vi "Tell.vi"(4 "Priority":bool, 6 "Self Attributes":refnum<class "Attributes.lvclass">, 8 "Relation":T1, 9 "Msg":refnum<class "Msg.lvclass">, 10 "Address":refnum<user-event>) -> (0 "Error out":errorcluster)   [LabVIEW 2025, in "jettl.lvlib" / "Actor.lvlib"]
uses:
  Actor.lvlib
  Msg/Msg.lvclass
  Attributes/Attributes/Attributes.lvclass
  Relation.ctl
  <vilib>/event_ctls.llb/usereventprio.ctl
  Teller/Teller.lvlib
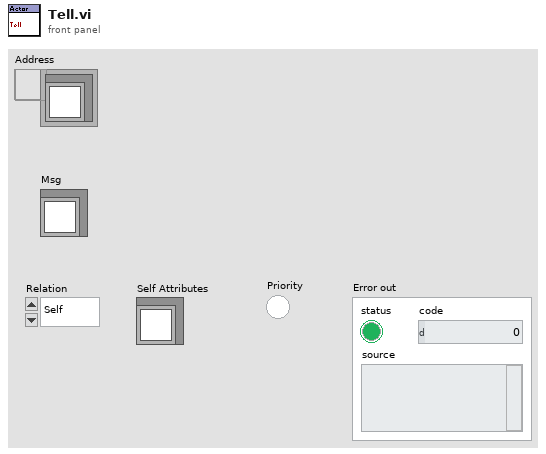
[diagram p1: front panel]
types:
  T1 = typedef "jettl.lvlib/Actor.lvlib/Relation.ctl" = enum16{"Self", "Parent", "Child"}
  T2 = typedef "usereventprio.ctl" = enum32{"high priority", "normal priority"}
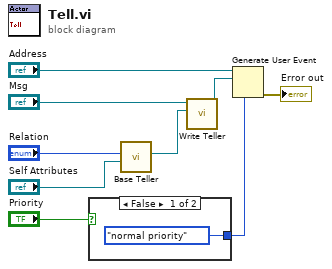
[diagram p0: block diagram]
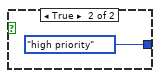
[diagram p2: hidden frame]
diagram:
  n1 = case shown="False" "Priority" {
    tunnel: [usereventprio."normal priority" ("priority (normal)") usereventprio."high priority" ("priority (normal)")] -> w9
    frame False {
    }
    frame True {
    }
  }
  n2 = call "Base Teller.vi"("Self Attributes"="Self Attributes", "Relation"="Relation") -> ("Teller"=w3:refnum<class "Teller.lvclass">)  [unwired: 9 in]
  n3 = call-dynamic "Write Teller.vi"("Teller"=w3, "Msg in"="Msg") -> ("Msg out"=w6:refnum<class "Msg.lvclass">)  [unwired: 9 in]
  n4 = Generate User Event(priority (normal)=w9, user event="Address", event data cluster=w6) -> (error out=→"Error out":errorcluster)  [unwired: 1 in, 1 out]
